vi "Claw Loop.vi"(8 "error in (no error)":errorcluster) -> ()   [LabVIEW 2014]
doc: "This VI runs in parallel to other tasks. It can contain as many user-defined periodic loops as you need. These can carry out PID or other sorts of timed response."
uses:
  Robot Global Data.vi
  <vilib>/Rock Robotics/Network Tables/SD Write Number.vi
panel:
  out "Claw State 2":dbl=2.0
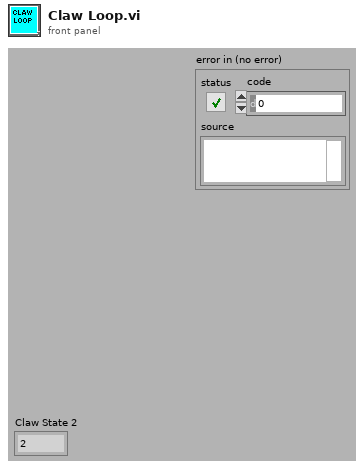
[diagram p1: front panel]
types:
  T1 = typedef "WPI_MotorControlDeviceRef.ctl" = cluster{"DeviceStatus":errorcluster, "Type":T2, "PWM":cluster{"Controller":T3, "PWM Channel":T4, "DeadBand":T5}, "CAN":cluster{"Device Number":u8, "Control Mode":T6, "Semaphore":T7, "Max Vout":dbl, "TalonSRX Control Mode":T8}, "Invert":bool, "TransformRef":T9, "InvTransformRef":T9}
  T2 = typedef "WPI_MotorControlType.ctl" = enum16{"PWM", "CAN", "CANTalonSRX"}
  T3 = typedef "FPGA_TypedefDigitalModule.ctl" = enum16{"Controller 1"}
  T4 = typedef "FPGA_DIOPWMChannel.ctl" = enum8{"PWM 0", "PWM 1", "PWM 2", "PWM 3", "PWM 4", "PWM 5", "PWM 6", "PWM 7", "PWM 8", "PWM 9", "PWM MXP 0", "PWM MXP 1", "PWM MXP 2", "PWM MXP 3", "PWM MXP 4", "PWM MXP 5", "PWM MXP 6", "PWM MXP 7", "PWM MXP 8", "PWM MXP 9", "Invalid"}
  T5 = typedef "WPI_PWMDeadband.ctl" = cluster{"Name":string, "maxPositivePwm":i32, "minPositivePwm":i32, "centerPwm":i32, "maxNegativePwm":i32, "minNegativePwm":i32, "angularRange":u16}
  T6 = typedef "WPI_CANJaguar_ControlMode.ctl" = enum8{"Percent VBus", "Current", "Speed", "Position", "Voltage"}
  T7 = typedef "Semaphore RefNum" = refnum<k1>
  T8 = typedef "WPI_CANTalonSRX_APIControlMode.ctl" = enum8{"Percent VBus", "Speed", "Position", "Slave", "Unchanged / Invalid"}
  T9 = typedef "WPI_PWMTransform_ConPane.ctl" = refnum<vi>
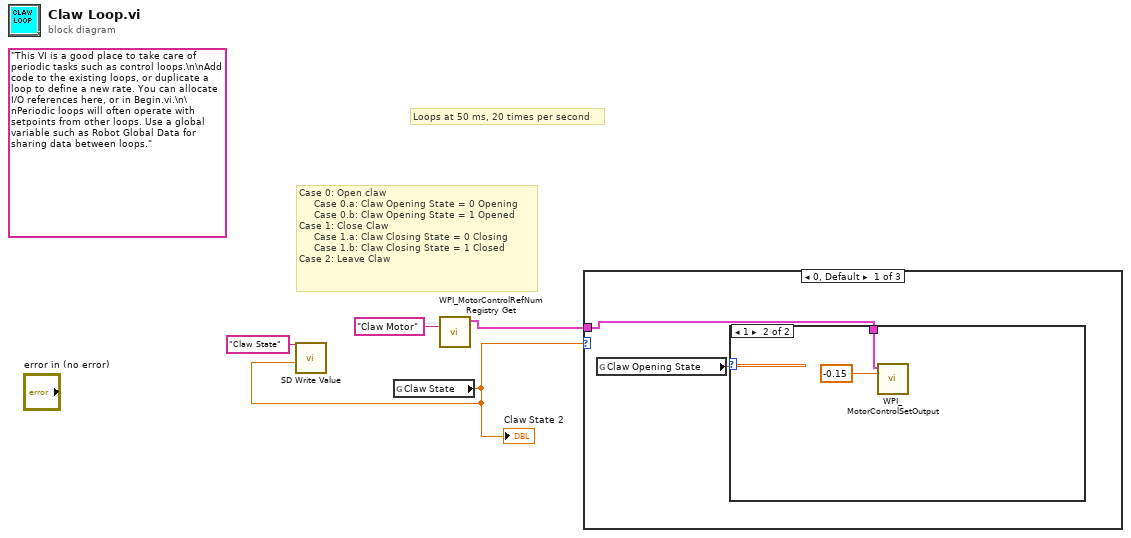
[diagram p0: block diagram]
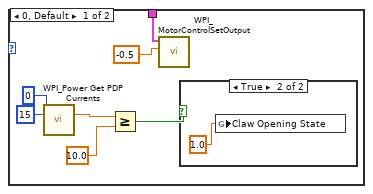
[diagram p2: hidden frame]
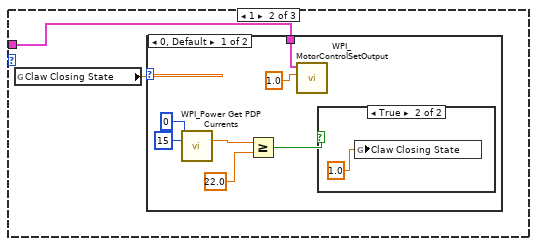
[diagram p4: hidden frame]
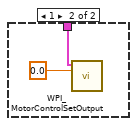
[diagram p6: hidden frame]
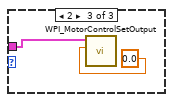
[diagram p7: hidden frame]
diagram:
  (unwired) "This VI is a good place to take care of periodic tasks such as control loops.\n\nAdd code to the existing loops, or duplicate a loop to define a new rate. You can allocate I/O references here, or in Begin.vi.\n\nPeriodic loops will often operate with setpoints from other loops. Use a global variable such as Robot Global Data for sharing data between loops."
  # "Case 0: Open claw\n     Case 0.a: Claw Opening State = 0 Opening\n     Case 0.b: Claw Opening State = 1 Opened\nCase 1: Close Claw \n     Case 1.a: Claw Closing State = 0 Closing\n     Case 1.b: Claw Closing State = 1 Closed\nCase 2: Leave Claw"
  # "Loops at 50 ms, 20 times per second"
  n1 = global read "Robot Global Data.vi" "Claw State"() -> (w1:dbl)
  "Claw State 2" <- w1
  n2 = call-poly <vilib>:"SD Write Value.vi"("Numeric"=w1, "Name"="Claw State") -> ()  [unwired: 8 in, 2 out]
  n3 = call <vilib>:"WPI_MotorControlRefNum Registry Get.vi"("refnum name"="Claw Motor") -> ("MotorControlDevRef"=w3:T1)  [unwired: 9 in, 1 out]
  n4 = case shown="0, Default" w1 {
    tunnel: w3 -> [w5 w18 w30]
    frame 0, Default {
      n5 = global read "Robot Global Data.vi" "Claw Opening State"() -> (w6:dbl)
      n6 = case shown="1" w6 {
        tunnel: w5 -> [w12 w15]
        frame 0, Default {
          n7 = call <vilib>:"WPI_Power Get PDP Currents.vi"("Power Distribution Panel (0)"=u8 0, "PDP Channel"=15) -> ("current (A)"=w8:dbl)  [unwired: 11 in, 2 out]
          n8 = Greater Or Equal?(x=w8, y=10.0) -> (x >= y?=w11:bool)
          n9 = call <vilib>:"WPI_MotorControlSetOutput.vi"("Output"=-0.5, "MotorControlDevRef"=w12) -> ()  [unwired: 7 in, 3 out]
          n10 = case shown="True" w11 {
            frame False {
            }
            frame True {
              n11 = global write "Robot Global Data.vi" "Claw Opening State"(1.0 ("y")) -> ()
            }
          }
        }
        frame 1 {
          n12 = call <vilib>:"WPI_MotorControlSetOutput.vi"("Output"=-0.15, "MotorControlDevRef"=w15) -> ()  [unwired: 7 in, 3 out]
        }
      }
    }
    frame 1 {
      n13 = global read "Robot Global Data.vi" "Claw Closing State"() -> (w17:dbl)
      n14 = case shown="0, Default" w17 {
        tunnel: w18 -> [w24 w27]
        frame 0, Default {
          n15 = call <vilib>:"WPI_Power Get PDP Currents.vi"("Power Distribution Panel (0)"=u8 0, "PDP Channel"=15) -> ("current (A)"=w20:dbl)  [unwired: 11 in, 2 out]
          n16 = Greater Or Equal?(x=w20, y=22.0) -> (x >= y?=w23:bool)
          n17 = call <vilib>:"WPI_MotorControlSetOutput.vi"("Output"=1.0, "MotorControlDevRef"=w24) -> ()  [unwired: 7 in, 3 out]
          n18 = case shown="True" w23 {
            frame False {
            }
            frame True {
              n19 = global write "Robot Global Data.vi" "Claw Closing State"(1.0 ("y")) -> ()
            }
          }
        }
        frame 1 {
          n20 = call <vilib>:"WPI_MotorControlSetOutput.vi"("Output"=0.0, "MotorControlDevRef"=w27) -> ()  [unwired: 7 in, 3 out]
        }
      }
    }
    frame 2 {
      n21 = call <vilib>:"WPI_MotorControlSetOutput.vi"("Output"=0.0, "MotorControlDevRef"=w30) -> ()  [unwired: 7 in, 3 out]
    }
  }
